vi "SaveToMemory.vi"(4 "error in (no error)":errorcluster, 6 "DeviceKey In":string, 7 "CmdLib In":refnum<k24>) -> (0 "error out":errorcluster, 2 "DeviceKey Out":string, 3 "CmdLib Out":refnum<k24>)   [LabVIEW 2013]
uses:
  C:/Users/Saffmanlab/Documents/git/CsPyController/labview/cesium_controller/PicoMotor/NewFocus8742/CmdLib.dll
  CmdLib.dll
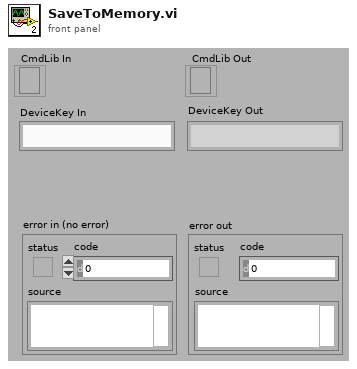
[diagram p1: front panel]
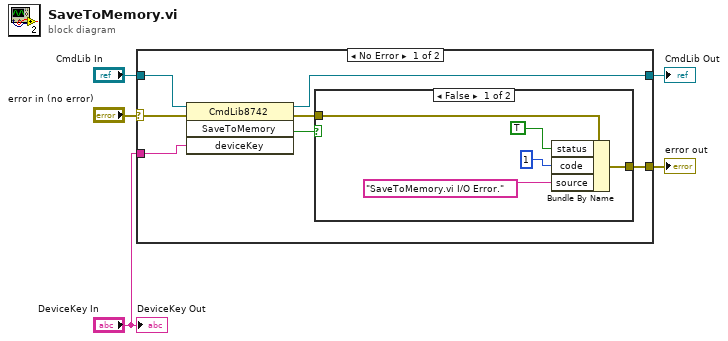
[diagram p0: block diagram]
diagram:
  n1 = case shown="No Error" "error in (no error)" {
    selector: "error in (no error)" -> [w9 w19]
    tunnel: "CmdLib In" -> [w12 w20]
    tunnel: [w11 w20] -> w4
    tunnel: "DeviceKey In" -> [w10 _]
    tunnel: [w6 w19] -> w1
    frame No Error {
      n2 = invoke class="CmdLib8742" method="SaveToMemory"(reference=w12, error in=w9, "deviceKey"=w10) -> (reference out=w11:refnum<k24>, error out=w7:errorcluster, "SaveToMemory"=w8:bool)  [unwired: 1 in, 1 out]
      n3 = case shown="False" w8 {
        tunnel: w7 -> [w17 w18]
        tunnel: [w16 w18] -> w6
        frame False {
          n4 = Bundle By Name(cluster=w17, "status"=TRUE, "code"=1, "source"="SaveToMemory.vi I/O Error.") -> (w16:errorcluster)
        }
        frame True {
        }
      }
    }
    frame Error {
    }
  }
  "error out" <- w1
  "CmdLib Out" <- w4
  "DeviceKey Out" <- "DeviceKey In"
